vi "CLN.vi"() -> ()   [LabVIEW 2020]
uses:
  myDll/Debug/myDll.dll
panel:
  out "Size":i32
  out "Sum":sgl
  in  "ptr":sgl[](array[numeric])
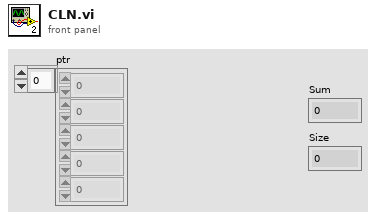
[diagram p1: front panel]
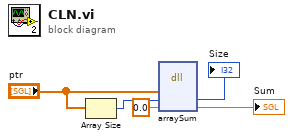
[diagram p0: block diagram]
diagram:
  n1 = Array Size(array="ptr") -> (size(s)=w4:i32)
  n2 = dll-call lib="C:/Users/Techie/Desktop/myDll/Debug/myDll.dll" fn="arraySum"("ptr"="ptr", "Size"=w4, "Sum"=sgl 0.0) -> ("Size"=→"Size":i32, "Sum"=→"Sum":sgl)  [unwired: 5 in, 2 out]
